vi "AutoIndicator.vi"(4 "i":i32, 5 "Neutral Zone":bool, 7 "2 Gear":bool, 8 "Alliance":enum16{"Blue", "Red"}(ring), 9 "2 Gear Side":enum16{"Left", "Right"}(ring), 10 "Tower Side":enum16{"Center", "Left", "Right"}(ring), 11 "Routine":enum16{"Gears", "Nothing", "Reach"}(ring)) -> (3 "Image":T1(plugin-control))   [LabVIEW 2016]
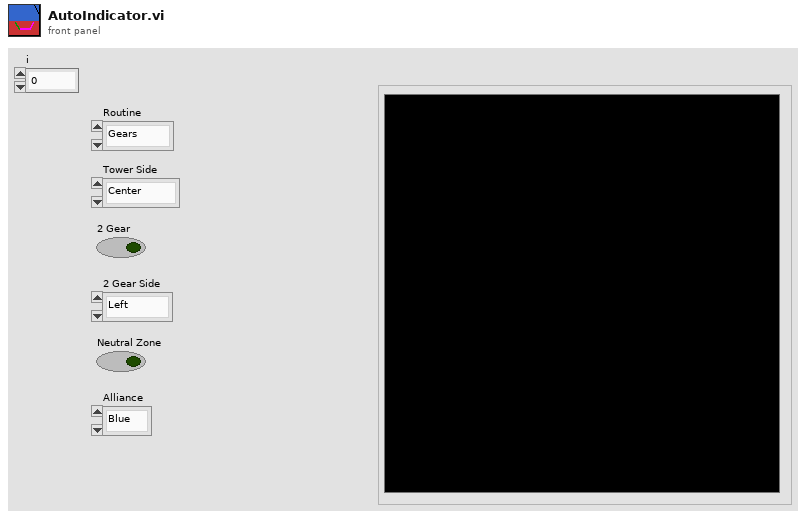
[diagram p1: front panel]
types:
  T1 = typedef "IMAQ Image.ctl" = refnum<image>
  T2 = cluster{"Left":i32, "Top":i32, "Right":i32, "Bottom":i32}
  T3 = typedef "Image Type" = u32
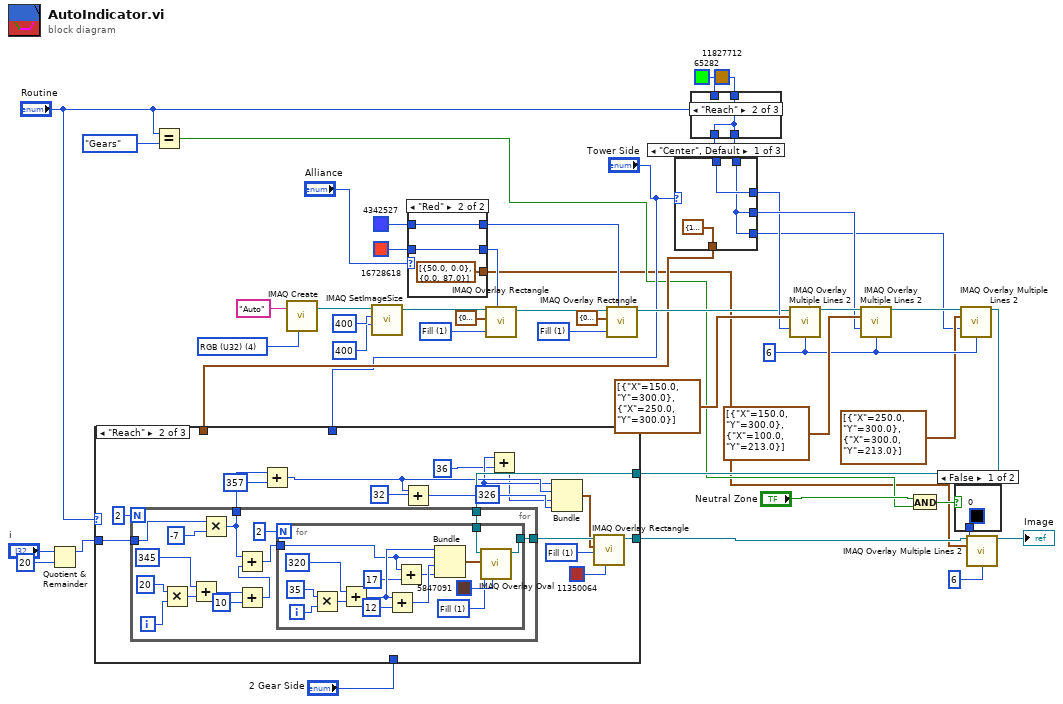
[diagram p0: block diagram]
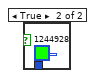
[diagram p2: hidden frame]
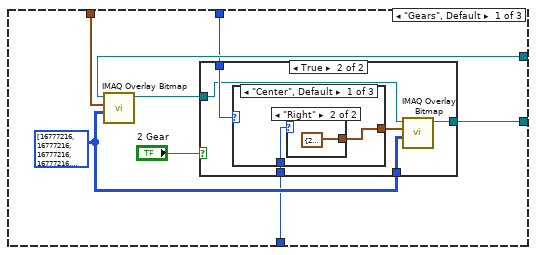
[diagram p3: hidden frame]
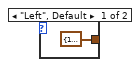
[diagram p5: hidden frame]
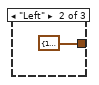
[diagram p6: hidden frame]
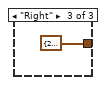
[diagram p7: hidden frame]
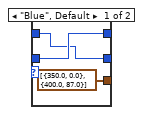
[diagram p11: hidden frame]
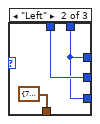
[diagram p12: hidden frame]
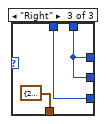
[diagram p13: hidden frame]
diagram:
  w27 = u32 1 items=["Frame", "Fill", "Highlight"] ("Drawing Mode (Frame)")
  w32 = u32 1 items=["Frame", "Fill", "Highlight"] ("Drawing Mode (Frame)")
  w38 = u32 6 ("Width")
  w46 = T3 4 items=["Grayscale (U8)", "Grayscale (I16)", "Grayscale (SGL)", "Complex (CSG)", "RGB (U32)", "HSL (U32)", "RGB (U64)", "Grayscale (U16)"] ("Image Type")
  n1 = Quotient & Remainder(x="i", y=20) -> (x-y*floor(x/y)=w8:i32)  [unwired: 1 out]
  n2 = Equal?(x="Routine", y=enum16{"Gears", "Nothing", "Reach"}."Gears") -> (x = y?=w3:bool)
  n3 = call "IMAQ Create"("Image Name"="Auto", "Image Type"=w46) -> ("New Image"=w45:T1)  [unwired: 3 in, 1 out]
  n4 = call "IMAQ SetImageSize"("Y Resolution"=400, "X Resolution"=400, "Image"=w45) -> ("Image Out"=w22:T1)  [unwired: 2 in, 1 out]
  n5 = case shown="\"Red\"" "Alliance" {
    tunnel: u32 4342527 ("Color") -> [w49 w52]
    tunnel: u32 16728618 ("Color") -> [w50 w53]
    tunnel: [w49 w53] -> w28
    tunnel: [w50 w52] -> w23
    tunnel: [cluster{"X":dbl, "Y":dbl}[] [{"X"=350.0, "Y"=0.0}, {"X"=400.0, "Y"=87.0}] ("Line End Points") cluster{"X":dbl, "Y":dbl}[] [{"X"=50.0, "Y"=0.0}, {"X"=0.0, "Y"=87.0}] ("Line End Points")] -> w2
    frame "Blue", Default {
    }
    frame "Red" {
    }
  }
  n6 = call "IMAQ Overlay Rectangle"("Color"=w28, "Drawing Mode (Frame)"=w32, "Rectangle"=T2 {"Left"=0, "Top"=400, "Right"=400, "Bottom"=200}, "Image"=w22) -> ("Image Out"=w25:T1)  [unwired: 6 in, 1 out]
  n7 = call "IMAQ Overlay Rectangle"("Color"=w23, "Drawing Mode (Frame)"=w27, "Rectangle"=T2 {"Left"=0, "Top"=0, "Right"=400, "Bottom"=200}, "Image"=w25) -> ("Image Out"=w24:T1)  [unwired: 6 in, 1 out]
  n8 = case shown="\"Reach\"" "Routine" {
    tunnel: [w55 w56 w57] -> w16
    tunnel: u32 11827712 ("Color") -> [w55 w56 w57]
    tunnel: [w54 w56 w57] -> w13
    tunnel: u32 65282 ("Color") -> [w54 _ _]
    frame "Gears", Default {
    }
    frame "Reach" {
    }
    frame "Nothing" {
    }
  }
  n9 = case shown="\"Center\", Default" "Tower Side" {
    tunnel: [w60 w62 w65] -> w35
    tunnel: [w59 w63 w65] -> w36
    tunnel: [w59 w62 w66] -> w34
    tunnel: w16 -> [w59 w62 w65]
    tunnel: w13 -> [w60 w63 w66]
    tunnel: [cluster{"X":i32, "Y":i32} {"X"=174, "Y"=300} ("Top Left Point 2") cluster{"X":i32, "Y":i32} {"X"=78, "Y"=250} ("Top Left Point 2") cluster{"X":i32, "Y":i32} {"X"=271, "Y"=250} ("Top Left Point 2")] -> w20
    frame "Center", Default {
    }
    frame "Left" {
    }
    frame "Right" {
    }
  }
  n10 = call "IMAQ Overlay Multiple Lines 2"("Image"=w24, "Line End Points"=cluster{"X":dbl, "Y":dbl}[] [{"X"=150.0, "Y"=300.0}, {"X"=250.0, "Y"=300.0}], "Color"=w35, "Width"=w38) -> ("Image Out"=w40:T1)  [unwired: 10 in, 1 out]
  n11 = call "IMAQ Overlay Multiple Lines 2"("Image"=w40, "Line End Points"=cluster{"X":dbl, "Y":dbl}[] [{"X"=150.0, "Y"=300.0}, {"X"=100.0, "Y"=213.0}], "Color"=w36, "Width"=w38) -> ("Image Out"=w39:T1)  [unwired: 10 in, 1 out]
  n12 = And(x="Neutral Zone", y=w3) -> (x .and. y?=w5:bool)
  n13 = case shown="False" w5 {
    tunnel: [u32 0 ("Color") u32 1244928 ("Color")] -> w10
    frame False {
    }
    frame True {
    }
  }
  n14 = call "IMAQ Overlay Multiple Lines 2"("Image"=w39, "Line End Points"=cluster{"X":dbl, "Y":dbl}[] [{"X"=250.0, "Y"=300.0}, {"X"=300.0, "Y"=213.0}], "Color"=w34, "Width"=w38) -> ("Image Out"=w21:T1)  [unwired: 10 in, 1 out]
  n15 = case shown="\"Reach\"" "Routine" {
    tunnel: w21 -> [w76 w105 w135]
    tunnel: w20 -> [w73 _ _]
    tunnel: [w72 w102 w135] -> w19
    tunnel: "Tower Side" -> [w71 _ _]
    tunnel: "2 Gear Side" -> [w69 _ _]
    tunnel: w8 -> [_ w103 _]
    frame "Gears", Default {
      w70 = u32[][] [[16777216, 16777216, 16777216, 16777216, 16777216, 16777216, 16777216, 16777216, 16777216, 16777216, 16777216, 16777216, 16777216, 16777216, 16777216, 16777216, 16777216, 16777216, 16777216, 16777216, 16777216, 16777216, 16777216, 16777216, 16777216, 16777216, 16777216, 16777216, 16777216, 16777216, 16777216, 16777216, 16777216, 16777216, 16777216, 16777216, 16777216, 16777216, 16777216, 16777216, 16777216, 16777216, 16777216, 16777216, 16777216, 16777216, 16777216, 16777216, 16777216, 16777216], [16777216, 16777216, 16777216, 16777216, 16777216, 16777216, 16777216, 16777216, 16777216, 16777216, 16777216, 16777216, 16777216, 16777216, 16777216, 16777216, 16777216, 16777216, 16777216, 16777216, 16777216, 16777216, 16777216, 16777216, 16777216, 16777216, 16777216, 16777216, 16777216, 16777216, 16777216, 16777216, 16777216, 16777216, 16777216, 16777216, 16777216, 16777216, 16777216, 16777216, 16777216, 16777216, 16777216, 16777216, 16777216, 16777216, 16777216, 16777216, 16777216, 16777216], [16777216, 16777216, 16777216, 16777216, 16777216, 16777216, 16777216, 16777216, 16777216, 16777216, 16777216, 16777216, 16777216, 16777216, 16777216, 16777216, 16777216, 16777216, 16777216, 16777216, 16777216, 16777216, 16777216, 16777216, 16777216, 16777216, 16777216, 16777216, 16777216, 16777216, 16777216, 16777216, 16777216, 16777216, 16777216, 16777216, 16777216, 16777216, 16777216, 16777216, 16777216, 16777216, 16777216, 16777216, 16777216, 16777216, 16777216, 16777216, 16777216, 16777216], [16777216, 16777216, 16777216, 16777216, 16777216, 16777216, 16777216, 16777216, 16777216, 16777216, 16777216, 16777216, 16777216, 16777216, 16777216, 16777216, 16777216, 16777216, 16777216, 16777216, 16777216, 16777216, 16777216, 16777216, 16777216, 16777216, 16777216, 16777216, 16777216, 16777216, 16777216, 16777216, 16777216, 16777216, 16777216, 16777216, 16777216, 16777216, 16777216, 16777216, 16777216, 16777216, 16777216, 16777216, 16777216, 16777216, 16777216, 16777216, 16777216, 16777216], [16777216, 16777216, 16777216, 16777216, 16777216, 16777216, 16777216, 16777216, 16777216, 16777216, 16777216, 16777216, 16777216, 16777216, 16777216, 16777216, 16777216, 16777216, 16777216, 16777216, 16777216, 16777216, 16777216, 16777216, 16777216, 16777216, 16777216, 16777216, 16777216, 16777216, 16777216, 16777216, 16777216, 16777216, 16777216, 16777216, 16777216, 16777216, 16777216, 16777216, 16777216, 16777216, 16777216, 16777216, 16777216, 16777216, 16777216, 16777216, 16777216, 16777216], [16777216, 16777216, 16777216, 16777216, 16777216, 16777216, 16777216, 16777216, 16777216, 16777216, 16777216, 16777216, 16777216, 16777216, 16777216, 16777216, 16777216, 16777216, 16777216, 16777216, 16777216, 16777216, 16777216, 16777216, 16777216, 16777216, 16777216, 16777216, 16777216, 16777216, 16777216, 16777216, 16777216, 16777216, 16777216, 16777216, 16777216, 16777216, 16777216, 16777216, 16777216, 16777216, 16777216, 16777216, 16777216, 16777216, 16777216, 16777216, 16777216, 16777216], [16777216, 16777216, 16777216, 16777216, 16777216, 16777216, 16777216, 16777216, 16777216, 16777216, 16777216, 16777216, 16777216, 16777216, 16777216, 16777216, 16777216, 16777216, 16777216, 16777216, 16777216, 16777216, 16777216, 16777216, 16777216, 16777216, 16777216, 16777216, 16777216, 16777216, 16777216, 16777216, 16777216, 16777216, 16777216, 16777216, 16777216, 16777216, 16777216, 16777216, 16777216, 16777216, 16777216, 16777216, 16777216, 16777216, 16777216, 16777216, 16777216, 16777216], [16777216, 16777216, 16777216, 16777216, 16777216, 16777216, 16777216, 16777216, 16777216, 16777216, 16777216, 16777216, 16777216, 16777216, 16777216, 16777216, 16777216, 13675604, 14724661, 15253036, 15187502, 15054879, 13616041, 16777216, 14395432, 14461485, 14987051, 14725940, 13741638, 13021574, 16777216, 16777216, 16777216, 16777216, 16777216, 16777216, 16777216, 16777216, 16777216, 16777216, 16777216, 16777216, 16777216, 16777216, 16777216, 16777216, 16777216, 16777216, 16777216, 16777216], [16777216, 16777216, 16777216, 16777216, 16777216, 16777216, 16777216, 16777216, 16777216, 16777216, 16777216, 16777216, 16777216, 16777216, 16777216, 16777216, 14133300, 12879886, 14199346, 15185952, 14791204, 14922529, 14857498, 16777216, 14658581, 14460961, 14395443, 16040509, 15976491, 15910701, 15582763, 15328211, 16777216, 16777216, 16777216, 16777216, 16777216, 16777216, 16777216, 16777216, 16777216, 16777216, 16777216, 16777216, 16777216, 16777216, 16777216, 16777216, 16777216, 16777216], [16777216, 16777216, 16777216, 16777216, 16777216, 16777216, 16777216, 16777216, 16777216, 16777216, 16777216, 16777216, 16777216, 16777216, 16777216, 16777216, 15383628, 12813824, 12750127, 14593063, 14196761, 14000410, 14263328, 14460707, 10970121, 14067016, 14527539, 16106300, 15582503, 15582504, 15450918, 15262158, 16777216, 16777216, 16777216, 16777216, 16777216, 16777216, 16777216, 16777216, 16777216, 16777216, 16777216, 16777216, 16777216, 16777216, 16777216, 16777216, 16777216, 16777216], [16777216, 16777216, 16777216, 16777216, 16777216, 16777216, 16777216, 16777216, 16777216, 16777216, 16777216, 16777216, 16777216, 16777216, 16777216, 16777216, 14593071, 11692037, 11297540, 14264359, 13999127, 14064411, 14065440, 14723352, 11495171, 11232527, 9261333, 15778592, 15450140, 15450401, 15384095, 16777216, 16777216, 16777216, 16777216, 16777216, 16777216, 16777216, 16777216, 16777216, 16777216, 16777216, 16777216, 16777216, 16777216, 16777216, 16777216, 16777216, 16777216, 16777216], [16777216, 16777216, 16777216, 16777216, 16777216, 16777216, 16777216, 16777216, 16777216, 16777216, 16777216, 16777216, 16777216, 16777216, 16777216, 16777216, 14395946, 12021505, 11298568, 14067232, 13999899, 13934365, 13736473, 15379994, 11758084, 12085516, 14527001, 15382804, 15252507, 15186205, 15120670, 16777216, 16777216, 16777216, 16777216, 16777216, 16777216, 16777216, 16777216, 16777216, 16777216, 16777216, 16777216, 16777216, 16777216, 16777216, 16777216, 16777216, 16777216, 16777216], [16777216, 16777216, 16777216, 16777216, 16777216, 16777216, 16777216, 16777216, 16777216, 16777216, 16777216, 16777216, 16777216, 16777216, 16777216, 16777216, 13870112, 14329626, 11627273, 14199328, 14461212, 14461212, 14329626, 14987546, 12018945, 13802793, 14854426, 14857225, 15054354, 14923033, 14923295, 16777216, 16777216, 16777216, 16777216, 16777216, 16777216, 16777216, 16777216, 16777216, 16777216, 16777216, 16777216, 16777216, 16777216, 16777216, 16777216, 16777216, 16777216, 16777216], [16777216, 16777216, 16777216, 16777216, 16777216, 16777216, 16777216, 16777216, 16777216, 16777216, 16777216, 13607720, 13607194, 12749580, 12025867, 11960339, 14001445, 13935895, 13935899, 13869591, 14001940, 14066452, 14133015, 14526490, 11296770, 14592536, 14788884, 15647008, 15713058, 15515683, 14924599, 16777216, 14592788, 14854930, 15977788, 15845951, 15583048, 16777216, 16777216, 16777216, 16777216, 16777216, 16777216, 16777216, 16777216, 16777216, 16777216, 16777216, 16777216, 16777216], [16777216, 16777216, 16777216, 16777216, 16777216, 16777216, 16777216, 16777216, 16777216, 16777216, 16777216, 13473553, 13475859, 13607194, 13012236, 12420366, 13935644, 14066193, 11234560, 10773504, 10839299, 10253105, 16777216, 16777216, 16777216, 14395415, 14395157, 15516182, 15515419, 15383833, 14789138, 14723085, 14196238, 14460685, 15844135, 16043065, 15846453, 15583302, 16777216, 16777216, 16777216, 16777216, 16777216, 16777216, 16777216, 16777216, 16777216, 16777216, 16777216, 16777216], [16777216, 16777216, 16777216, 16777216, 16777216, 16777216, 16777216, 16777216, 16777216, 16777216, 14002745, 13540886, 7218688, 8732948, 13738520, 13672725, 13935382, 12287236, 11958021, 12155652, 12221704, 16777216, 16777216, 16777216, 16777216, 16777216, 14329877, 14723606, 15513622, 14723602, 13933064, 9784066, 14855192, 11101193, 14789138, 16174648, 15846200, 15583040, 15385921, 16777216, 16777216, 16777216, 16777216, 16777216, 16777216, 16777216, 16777216, 16777216, 16777216, 16777216], [16777216, 16777216, 16777216, 16777216, 16777216, 16777216, 16777216, 16777216, 16777216, 16777216, 16777216, 14132765, 10968578, 10049280, 13672987, 13804309, 13869589, 14789916, 12483586, 12088578, 12354070, 12750630, 16777216, 16777216, 16777216, 15658475, 14264852, 14592018, 14526741, 14723602, 9783552, 11099399, 8075265, 14854930, 14723344, 15318041, 14463522, 14003495, 13806129, 16777216, 16777216, 16777216, 16777216, 16777216, 16777216, 16777216, 16777216, 16777216, 16777216, 16777216], [16777216, 16777216, 16777216, 16777216, 16777216, 16777216, 16777216, 16777216, 16777216, 16777216, 16777216, 16777216, 14459923, 13406238, 10704640, 11367953, 11236625, 13935634, 13339395, 12681994, 12551449, 12749341, 16777216, 16777216, 16777216, 14395670, 14526223, 11696926, 14329613, 14592786, 11889156, 11362561, 11496970, 14526478, 14920721, 13344295, 13147437, 12950325, 16777216, 16777216, 16777216, 16777216, 16777216, 16777216, 16777216, 16777216, 16777216, 16777216, 16777216, 16777216], [16777216, 16777216, 16777216, 16777216, 16777216, 16777216, 16777216, 16777216, 16777216, 16777216, 16777216, 16777216, 13475608, 13606934, 12946944, 11498762, 11170056, 13935382, 14855706, 13077265, 12880412, 12815130, 13079070, 16777216, 14264872, 14329614, 12156676, 11565340, 10316311, 14460432, 14127894, 13010717, 14789916, 14461453, 12555310, 12555821, 12358206, 16777216, 16777216, 16777216, 16777216, 16777216, 16777216, 16777216, 16777216, 16777216, 16777216, 16777216, 16777216, 16777216], [16777216, 16777216, 16777216, 16777216, 16777216, 16777216, 16777216, 16777216, 16777216, 16777216, 16777216, 16777216, 16777216, 13606671, 11958794, 11630348, 11958543, 12025365, 13935889, 13669651, 13078043, 13012250, 13078556, 16777216, 14263823, 14395407, 11565594, 11368476, 11434269, 14461202, 14658830, 14789135, 14592269, 12685068, 11962416, 11832390, 16777216, 16777216, 16777216, 16777216, 16777216, 16777216, 16777216, 16777216, 16777216, 16777216, 16777216, 16777216, 16777216, 16777216], [16777216, 16777216, 16777216, 16777216, 16777216, 16777216, 16777216, 16777216, 16777216, 16777216, 16777216, 16777216, 16777216, 13739021, 12155913, 11761933, 12287759, 11499791, 13869841, 14658578, 13209112, 13012763, 12946970, 14197778, 14263053, 11762458, 11631133, 11959323, 11894810, 16777216, 14723344, 15118864, 13935369, 14067733, 14199328, 16777216, 16777216, 16777216, 16777216, 16777216, 16777216, 16777216, 16777216, 16777216, 16777216, 16777216, 16777216, 16777216, 16777216, 16777216], [16777216, 16777216, 16777216, 16777216, 16777216, 16777216, 16777216, 16777216, 16777216, 16777216, 13738005, 13935895, 13541652, 14262801, 12221451, 12090378, 12353039, 13278266, 16579838, 14197260, 13537816, 13208599, 13541388, 14197260, 13800463, 11893278, 11894298, 11959837, 16777216, 16777216, 14592785, 15581726, 15120159, 15186213, 15120933, 16777216, 16777216, 16777216, 16777216, 16777216, 16777216, 16777216, 16777216, 16777216, 16777216, 16777216, 16777216, 16777216, 16777216, 16777216], [16777216, 16777216, 16777216, 16777216, 16777216, 16777216, 16777216, 16777216, 16777216, 13474066, 13212184, 12882457, 13475598, 13208840, 12353292, 12419085, 12485136, 16777216, 16777216, 13935887, 14921759, 13406232, 14132237, 14132494, 11890946, 11958293, 12024603, 16777216, 16777216, 16777216, 14526995, 15450704, 15449635, 15318564, 15318053, 14596674, 16777216, 16777216, 16777216, 16777216, 16777216, 16777216, 16777216, 16777216, 16777216, 16777216, 16777216, 16777216, 16777216, 16777216], [16777216, 16777216, 16777216, 16777216, 16777216, 16777216, 16777216, 16777216, 16777216, 13078543, 12747271, 10642178, 13344010, 13011461, 12418570, 12353805, 12550671, 16777216, 16777216, 16777216, 13537818, 11036427, 14066444, 12285187, 11889920, 12087810, 12091676, 16777216, 16777216, 16777216, 13740060, 14658062, 15185930, 15119632, 14528535, 14201439, 13742179, 13809009, 14400884, 16777216, 16777216, 16777216, 16777216, 16777216, 16777216, 16777216, 16777216, 16777216, 16777216, 16777216], [16777216, 16777216, 16777216, 16777216, 16777216, 16777216, 16777216, 16777216, 16777216, 14067996, 13275925, 8930560, 13475596, 13273606, 12484363, 12551184, 12812814, 16777216, 16777216, 16777216, 11824128, 11693577, 14592020, 13010707, 13207568, 13405970, 13209892, 16777216, 16777216, 16777216, 16777216, 14592010, 14657551, 14658062, 14854667, 15249937, 15778602, 15187782, 15055942, 15056453, 14990654, 16777216, 16777216, 16777216, 16777216, 16777216, 16777216, 16777216, 16777216, 16777216], [16777216, 16777216, 16777216, 16777216, 16777216, 16777216, 16777216, 16777216, 16777216, 16777216, 13605903, 13475596, 13737489, 13866503, 12944136, 12616201, 13538580, 13935117, 13935115, 14066444, 12487705, 11825414, 11499264, 15118362, 13207044, 12877827, 12749090, 12487472, 12554294, 16777216, 16777216, 14461451, 14394890, 8470023, 8405780, 14196488, 14526474, 15314968, 14856991, 14660131, 14331433, 16777216, 16777216, 16777216, 16777216, 16777216, 16777216, 16777216, 16777216, 16777216], [16777216, 16777216, 16777216, 16777216, 16777216, 16777216, 16777216, 16777216, 16777216, 16777216, 16777216, 16777216, 13409292, 13870354, 13672717, 13607181, 13868813, 13935887, 13870094, 13277965, 13733385, 12021505, 14132235, 14263051, 14329613, 14590476, 12947755, 13078328, 12947504, 12815920, 11898157, 12020742, 11824138, 11036688, 11760411, 14395658, 14394380, 14986768, 14462501, 14462752, 13805869, 16777216, 16777216, 16777216, 16777216, 16777216, 16777216, 16777216, 16777216, 16777216], [16777216, 16777216, 16777216, 16777216, 16777216, 16777216, 16777216, 16777216, 16777216, 16777216, 16777216, 16777216, 16777216, 13344523, 13607184, 13672723, 9656320, 9065219, 16777216, 16777216, 13804563, 14198027, 12353037, 10117888, 14066955, 14395407, 14723342, 13605164, 12881711, 12620089, 12093476, 14593039, 14788627, 11296770, 11629077, 14526474, 14264074, 14921232, 14396707, 13937188, 13674283, 16777216, 16777216, 16777216, 16777216, 16777216, 16777216, 16777216, 16777216, 16777216], [16777216, 16777216, 16777216, 16777216, 16777216, 16777216, 16777216, 16777216, 16777216, 16777216, 16777216, 16777216, 16777216, 13475596, 12221441, 11958021, 12023815, 12419345, 16777216, 16777216, 13870353, 14001931, 12419345, 12287761, 10183185, 14263569, 14395919, 14461199, 14789395, 12948533, 13803282, 14395660, 15250967, 14394629, 11626755, 14460935, 14329099, 15183895, 13871141, 13213478, 13082414, 16777216, 16777216, 16777216, 16777216, 16777216, 16777216, 16777216, 16777216, 16777216], [16777216, 16777216, 16777216, 16777216, 16777216, 16777216, 16777216, 16777216, 16777216, 16777216, 16777216, 16777216, 13344271, 13475596, 13208322, 12221956, 12025355, 12485906, 12749337, 16777216, 13804814, 14328844, 12485138, 12353554, 12354068, 10710034, 16777216, 14460430, 14395407, 14461459, 14526993, 14395919, 14526992, 14592269, 14526474, 14657551, 14657552, 15120700, 16777216, 16777216, 16777216, 16777216, 16777216, 16777216, 16777216, 16777216, 16777216, 16777216, 16777216, 16777216], [16777216, 16777216, 16777216, 16777216, 16777216, 16777216, 16777216, 16777216, 16777216, 16777216, 16777216, 13410064, 8931329, 9193748, 10969088, 13142278, 12486157, 12550929, 12683798, 16777216, 14000910, 14329099, 12420113, 12287761, 12485654, 12617751, 16777216, 16777216, 16777216, 14133518, 14395407, 13539094, 11895067, 11435310, 10251298, 16777216, 16777216, 16777216, 16777216, 16777216, 16777216, 16777216, 16777216, 16777216, 16777216, 16777216, 16777216, 16777216, 16777216, 16777216], [16777216, 16777216, 16777216, 16777216, 16777216, 16777216, 16777216, 16777216, 16777216, 16777216, 16777216, 12422656, 8796928, 10116867, 13607182, 13473024, 12879371, 12683536, 12551698, 12683797, 14000908, 14001678, 12550671, 12353039, 12550933, 12486165, 16777216, 16777216, 16777216, 16777216, 14395920, 12223511, 12091674, 12091938, 12421411, 16777216, 16777216, 16777216, 16777216, 16777216, 16777216, 16777216, 16777216, 16777216, 16777216, 16777216, 16777216, 16777216, 16777216, 16777216], [16777216, 16777216, 16777216, 16777216, 16777216, 16777216, 16777216, 16777216, 16777216, 16777216, 16777216, 13605649, 13606417, 8733449, 13541389, 13738510, 13077255, 12879886, 12288526, 12486419, 13935889, 14263820, 12615951, 12353041, 12485908, 12420115, 16777216, 16777216, 16777216, 14329875, 14329614, 13932296, 12748038, 12749077, 13080360, 13607718, 16777216, 16777216, 16777216, 16777216, 16777216, 16777216, 16777216, 16777216, 16777216, 16777216, 16777216, 16777216, 16777216, 16777216], [16777216, 16777216, 16777216, 16777216, 16777216, 16777216, 16777216, 16777216, 16777216, 16777216, 16777216, 13605903, 13080327, 13278217, 11040804, 13278773, 14131983, 13143822, 12682509, 12552212, 13804814, 14329614, 12549127, 12352779, 12419347, 12748561, 16777216, 16777216, 13740325, 14198289, 13343497, 14330380, 14394629, 14001427, 14001950, 13870364, 14002215, 16777216, 16777216, 16777216, 16777216, 16777216, 16777216, 16777216, 16777216, 16777216, 16777216, 16777216, 16777216, 16777216], [16777216, 16777216, 16777216, 16777216, 16777216, 16777216, 16777216, 16777216, 16777216, 16777216, 16777216, 16777216, 11969654, 16777216, 16777216, 16777216, 13804048, 14132496, 13012499, 12224274, 13935887, 14263821, 12483586, 12482560, 12615685, 13340688, 16777216, 13806129, 14264080, 14263053, 8732417, 9457680, 14592271, 14658838, 14461475, 14001949, 14133286, 15319894, 16777216, 16777216, 16777216, 16777216, 16777216, 16777216, 16777216, 16777216, 16777216, 16777216, 16777216, 16777216], [16777216, 16777216, 16777216, 16777216, 16777216, 16777216, 16777216, 16777216, 16777216, 16777216, 16777216, 16777216, 16777216, 16777216, 16777216, 16777216, 13475605, 13738767, 13738510, 13541129, 13870353, 14264334, 12680448, 13011470, 12813313, 12418820, 14330126, 14395409, 14329867, 14264074, 11100161, 11299086, 10582020, 14855958, 14593314, 14396961, 14002466, 13870890, 16777216, 16777216, 16777216, 16777216, 16777216, 16777216, 16777216, 16777216, 16777216, 16777216, 16777216, 16777216], [16777216, 16777216, 16777216, 16777216, 16777216, 16777216, 16777216, 16777216, 16777216, 16777216, 16777216, 16777216, 16777216, 16777216, 16777216, 16777216, 13672717, 9455616, 7153152, 13804301, 14000908, 14066701, 14461713, 14394637, 14132748, 14001932, 14198028, 11828480, 13540108, 14791198, 11627525, 11168013, 14198541, 14264334, 15185184, 14330655, 13870364, 12163157, 16777216, 16777216, 16777216, 16777216, 16777216, 16777216, 16777216, 16777216, 16777216, 16777216, 16777216, 16777216], [16777216, 16777216, 16777216, 16777216, 16777216, 16777216, 16777216, 16777216, 16777216, 16777216, 16777216, 16777216, 16777216, 16777216, 16777216, 16777216, 14001680, 9851392, 9390848, 13672975, 10380544, 14002193, 14067473, 14330645, 13936396, 14132748, 12814095, 12616464, 12222995, 14264084, 15249946, 14067982, 11231747, 14461713, 14526992, 12030272, 12033125, 16777216, 16777216, 16777216, 16777216, 16777216, 16777216, 16777216, 16777216, 16777216, 16777216, 16777216, 16777216, 16777216], [16777216, 16777216, 16777216, 16777216, 16777216, 16777216, 16777216, 16777216, 16777216, 16777216, 16777216, 16777216, 16777216, 16777216, 16777216, 16777216, 13540357, 10246912, 11102469, 13935887, 10444800, 9920266, 13935887, 14001680, 10574597, 13541129, 13670144, 12747789, 12617745, 11697429, 14002193, 14593298, 13737477, 14264080, 11965776, 11507812, 16777216, 16777216, 16777216, 16777216, 16777216, 16777216, 16777216, 16777216, 16777216, 16777216, 16777216, 16777216, 16777216, 16777216], [16777216, 16777216, 16777216, 16777216, 16777216, 16777216, 16777216, 16777216, 16777216, 16777216, 16777216, 16777216, 16777216, 16777216, 16777216, 16777216, 14331418, 11168001, 13344010, 12355328, 10446869, 9724441, 13409805, 12220424, 10838017, 8933382, 14461712, 12814356, 12355600, 12551958, 11048308, 16777216, 14133268, 12032347, 16777216, 16777216, 16777216, 16777216, 16777216, 16777216, 16777216, 16777216, 16777216, 16777216, 16777216, 16777216, 16777216, 16777216, 16777216, 16777216], [16777216, 16777216, 16777216, 16777216, 16777216, 16777216, 16777216, 16777216, 16777216, 16777216, 16777216, 16777216, 16777216, 16777216, 16777216, 16777216, 16777216, 13935117, 13803278, 11038996, 9395989, 16777216, 16777216, 14526225, 11035136, 10707462, 14132747, 12748559, 12420626, 12223765, 11901036, 16777216, 16777216, 16777216, 16777216, 16777216, 16777216, 16777216, 16777216, 16777216, 16777216, 16777216, 16777216, 16777216, 16777216, 16777216, 16777216, 16777216, 16777216, 16777216], [16777216, 16777216, 16777216, 16777216, 16777216, 16777216, 16777216, 16777216, 16777216, 16777216, 16777216, 16777216, 16777216, 16777216, 16777216, 16777216, 16777216, 16777216, 16777216, 16777216, 16777216, 16777216, 16777216, 13935115, 14000908, 14066444, 14198287, 12617745, 12026386, 11830042, 16777216, 16777216, 16777216, 16777216, 16777216, 16777216, 16777216, 16777216, 16777216, 16777216, 16777216, 16777216, 16777216, 16777216, 16777216, 16777216, 16777216, 16777216, 16777216, 16777216], [16777216, 16777216, 16777216, 16777216, 16777216, 16777216, 16777216, 16777216, 16777216, 16777216, 16777216, 16777216, 16777216, 16777216, 16777216, 16777216, 16777216, 16777216, 16777216, 16777216, 16777216, 16777216, 16777216, 15917232, 14461459, 14198287, 13936139, 12354833, 14931661, 16777216, 16777216, 16777216, 16777216, 16777216, 16777216, 16777216, 16777216, 16777216, 16777216, 16777216, 16777216, 16777216, 16777216, 16777216, 16777216, 16777216, 16777216, 16777216, 16777216, 16777216], [16777216, 16777216, 16777216, 16777216, 16777216, 16777216, 16777216, 16777216, 16777216, 16777216, 16777216, 16777216, 16777216, 16777216, 16777216, 16777216, 16777216, 16777216, 16777216, 16777216, 16777216, 16777216, 16777216, 16777216, 15526121, 16777216, 16777216, 16777216, 16777216, 16777216, 16777216, 16777216, 16777216, 16777216, 16777216, 16777216, 16777216, 16777216, 16777216, 16777216, 16777216, 16777216, 16777216, 16777216, 16777216, 16777216, 16777216, 16777216, 16777216, 16777216], [16777216, 16777216, 16777216, 16777216, 16777216, 16777216, 16777216, 16777216, 16777216, 16777216, 16777216, 16777216, 16777216, 16777216, 16777216, 16777216, 16777216, 16777216, 16777216, 16777216, 16777216, 16777216, 16777216, 16777216, 16777216, 16777216, 16777216, 16777216, 16777216, 16777216, 16777216, 16777216, 16777216, 16777216, 16777216, 16777216, 16777216, 16777216, 16777216, 16777216, 16777216, 16777216, 16777216, 16777216, 16777216, 16777216, 16777216, 16777216, 16777216, 16777216], [16777216, 16777216, 16777216, 16777216, 16777216, 16777216, 16777216, 16777216, 16777216, 16777216, 16777216, 16777216, 16777216, 16777216, 16777216, 16777216, 16777216, 16777216, 16777216, 16777216, 16777216, 16777216, 16777216, 16777216, 16777216, 16777216, 16777216, 16777216, 16777216, 16777216, 16777216, 16777216, 16777216, 16777216, 16777216, 16777216, 16777216, 16777216, 16777216, 16777216, 16777216, 16777216, 16777216, 16777216, 16777216, 16777216, 16777216, 16777216, 16777216, 16777216], [16777216, 16777216, 16777216, 16777216, 16777216, 16777216, 16777216, 16777216, 16777216, 16777216, 16777216, 16777216, 16777216, 16777216, 16777216, 16777216, 16777216, 16777216, 16777216, 16777216, 16777216, 16777216, 16777216, 16777216, 16777216, 16777216, 16777216, 16777216, 16777216, 16777216, 16777216, 16777216, 16777216, 16777216, 16777216, 16777216, 16777216, 16777216, 16777216, 16777216, 16777216, 16777216, 16777216, 16777216, 16777216, 16777216, 16777216, 16777216, 16777216, 16777216], [16777216, 16777216, 16777216, 16777216, 16777216, 16777216, 16777216, 16777216, 16777216, 16777216, 16777216, 16777216, 16777216, 16777216, 16777216, 16777216, 16777216, 16777216, 16777216, 16777216, 16777216, 16777216, 16777216, 16777216, 16777216, 16777216, 16777216, 16777216, 16777216, 16777216, 16777216, 16777216, 16777216, 16777216, 16777216, 16777216, 16777216, 16777216, 16777216, 16777216, 16777216, 16777216, 16777216, 16777216, 16777216, 16777216, 16777216, 16777216, 16777216, 16777216], [16777216, 16777216, 16777216, 16777216, 16777216, 16777216, 16777216, 16777216, 16777216, 16777216, 16777216, 16777216, 16777216, 16777216, 16777216, 16777216, 16777216, 16777216, 16777216, 16777216, 16777216, 16777216, 16777216, 16777216, 16777216, 16777216, 16777216, 16777216, 16777216, 16777216, 16777216, 16777216, 16777216, 16777216, 16777216, 16777216, 16777216, 16777216, 16777216, 16777216, 16777216, 16777216, 16777216, 16777216, 16777216, 16777216, 16777216, 16777216, 16777216, 16777216], [16777216, 16777216, 16777216, 16777216, 16777216, 16777216, 16777216, 16777216, 16777216, 16777216, 16777216, 16777216, 16777216, 16777216, 16777216, 16777216, 16777216, 16777216, 16777216, 16777216, 16777216, 16777216, 16777216, 16777216, 16777216, 16777216, 16777216, 16777216, 16777216, 16777216, 16777216, 16777216, 16777216, 16777216, 16777216, 16777216, 16777216, 16777216, 16777216, 16777216, 16777216, 16777216, 16777216, 16777216, 16777216, 16777216, 16777216, 16777216, 16777216, 16777216]] ("Array")
      n16 = call "IMAQ Overlay Bitmap"("Bitmap"=w70, "Top Left Point"=w73, "Image"=w76) -> ("Image Out"=w74:T1)  [unwired: 7 in, 1 out]
      n17 = case shown="True" "2 Gear" {
        tunnel: [w77 w83] -> w72
        tunnel: w74 -> [w77 w81]
        tunnel: w71 -> [_ w82]
        tunnel: w70 -> [_ w80]
        tunnel: w69 -> [_ w78]
        frame False {
        }
        frame True {
          n18 = case shown="\"Center\", Default" w82 {
            tunnel: [w84 cluster{"X":i32, "Y":i32} {"X"=125, "Y"=347} ("Top Left Point 2") cluster{"X":i32, "Y":i32} {"X"=230, "Y"=347} ("Top Left Point 2")] -> w79
            tunnel: w78 -> [w85 _ _]
            frame "Center", Default {
              n19 = case shown="\"Right\"" w85 {
                tunnel: [cluster{"X":i32, "Y":i32} {"X"=125, "Y"=347} ("Top Left Point 2") cluster{"X":i32, "Y":i32} {"X"=230, "Y"=347} ("Top Left Point 2")] -> w84
                frame "Left", Default {
                }
                frame "Right" {
                }
              }
            }
            frame "Left" {
            }
            frame "Right" {
            }
          }
          n20 = call "IMAQ Overlay Bitmap"("Bitmap"=w80, "Top Left Point"=w79, "Image"=w81) -> ("Image Out"=w83:T1)  [unwired: 7 in, 1 out]
        }
      }
    }
    frame "Reach" {
      w94 = 326 ("y")
      w90 = u32 1 items=["Frame", "Fill", "Highlight"] ("Drawing Mode (Frame)")
      n21 = for {
        N: 2 -> [_]
        tunnel: w105 -> [w113]
        tunnel: [w112] -> w101
        tunnel: w103 -> [w108]
        tunnel: [w106] -> w100
        i -> [w114]
        n22 = Multiply(x=20, y=w114) -> (x*y=w116:i32)
        n23 = Add(x=345, y=w116) -> (x+y=w119:i32)
        n24 = Multiply(x=w108, y=-7) -> (x*y=w106:i32)
        n25 = Add(x=w119, y=10) -> (x+y=w110:i32)
        n26 = Add(x=w106, y=w110) -> (x+y=w109:i32)
        n27 = for {
          N: 2 -> [_]
          tunnel: w109 -> [w123]
          tunnel: w113 -> [w127]
          tunnel: [w126] -> w112
          i -> [w132]
          w125 = u32 1 items=["Frame", "Fill"] ("Drawing Mode (Frame)")
          n28 = Multiply(x=35, y=w132) -> (x*y=w130:i32)
          n29 = Add(x=320, y=w130) -> (x+y=w128:i32)
          n30 = Add(x=w128, y=12) -> (x+y=w129:i32)
          n31 = Add(x=w123, y=17) -> (x+y=w124:i32)
          n32 = Bundle(w128, w123, w129, w124) -> (w133:cluster{i32, i32, i32, i32})  [unwired: 1 in]
          n33 = call "IMAQ Overlay Oval"("Color"=u32 5847091, "Drawing Mode (Frame)"=w125, "Bounding Rectangle"=w133, "Image"=w127) -> ("Image Out"=w126:T1)  [unwired: 6 in, 1 out]
        }
      }
      n34 = Add(x=w100, y=357 ("y 2")) -> (x+y=w95:i32)
      n35 = Add(x=w95, y=32 ("y 3")) -> (x+y=w96:i32)
      n36 = Add(x=w94, y=36 ("y 4")) -> (x+y=w93:i32)
      n37 = Bundle("y"=w94, w95, w93, w96) -> (w91:cluster{"y":i32, i32, i32, i32})  [unwired: 1 in]
      n38 = call "IMAQ Overlay Rectangle"("Color"=u32 11350064, "Drawing Mode (Frame)"=w90, "Rectangle"=w91, "Image"=w101) -> ("Image Out"=w102:T1)  [unwired: 6 in, 1 out]
    }
    frame "Nothing" {
    }
  }
  n39 = call "IMAQ Overlay Multiple Lines 2"("Image"=w19, "Line End Points"=w2, "Color"=w10, "Width"=u32 6) -> ("Image Out"=→"Image":T1)  [unwired: 10 in, 1 out]
